vi "toNextMonth.vi"(11 "Cron in":T1) -> (3 "Cron out":T1)   [LabVIEW 2013, in "openCron.lvlib" / "Cron.lvclass"]
uses:
  Cron.lvclass
  CronTime -- cluster.ctl
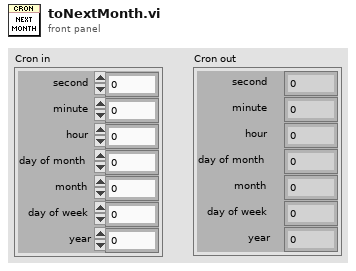
[diagram p1: front panel]
types:
  T1 = typedef "openCron.lvlib/Cron.lvclass/CronTime -- cluster.ctl" = cluster{"second":i32, "minute":i32, "hour":i32, "day of month":i32, "month":i32, "day of week":i32, "year":i32}
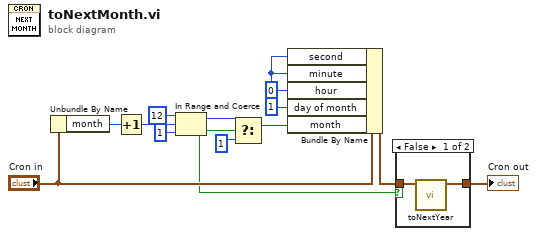
[diagram p0: block diagram]
diagram:
  w5 = 0 ("hour")
  n1 = Unbundle By Name("Cron in") -> ("month"=w13:i32)
  n2 = Increment(x=w13) -> (x+1=w10:i32)
  n3 = In Range and Coerce(upper limit=12, x=w10, lower limit=1) -> (coerced(x)=w8:i32, In Range?=w1:bool)
  n4 = Select(t=w8, s=w1, f=1 ("month")) -> (s? t:f=w11:i32)
  n5 = Bundle By Name(cluster="Cron in", "second"=w5, "minute"=w5, "hour"=w5, "day of month"=1 ("month"), "month"=w11) -> (w3:T1)
  n6 = case shown="False" w1 {
    tunnel: w3 -> [w15 w16]
    tunnel: [w14 w16] -> w2
    frame False {
      n7 = call "toNextYear.vi"("Cron in"=w15) -> ("Cron out"=w14:T1)  [unwired: 10 in]
    }
    frame True {
    }
  }
  "Cron out" <- w2
